vi "HAL camera start acquire.vi"(1 "error in":errorcluster) -> (0 "error out":errorcluster)   [LabVIEW 2011]
doc: "Starts an iXon acquisition (if not already running)"
uses:
  Cascade-specific globals.vi
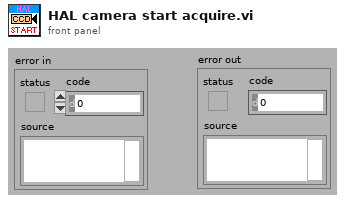
[diagram p1: front panel]
types:
  T1 = cluster{"Camera Handle":u32, "Pulser Handle":u32, "File Handle":u32, "Display Handle":u32, "Image Handle":u32}
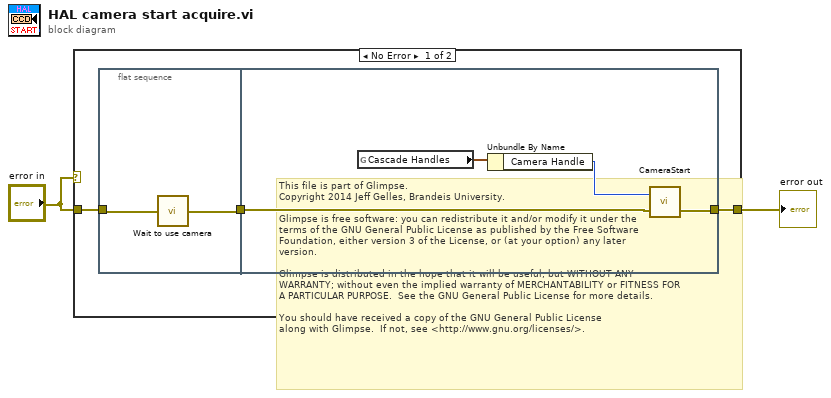
[diagram p0: block diagram]
diagram:
  # "This file is part of Glimpse. \nCopyright 2014 Jeff Gelles, Brandeis University.    \n\nGlimpse is free software: you can redistribute it and/or modify it under the \nterms of the GNU General Public License as published by the Free Software \nFoundation, either version 3 of the License, or (at your option) any later \nversion.\n\nGlimpse is distributed in the hope that it will be useful, but WITHOUT ANY \nWARRANTY; without even the implied warranty of MERCHANTABILITY or FITNESS FOR \nA PARTICULAR PURPOSE.  See the GNU General Public License for more details.\n\nYou should have received a copy of the GNU General Public License\nalong with Glimpse.  If not, see <http://www.gnu.org/licenses/>."
  n1 = case shown="No Error" "error in" {
    tunnel: "error in" -> [w5 w12]
    tunnel: [w4 w12] -> w2
    frame No Error {
      n2 = flat-sequence {
        tunnel: w5 -> [w6]
        tunnel: [w7] -> w3
        tunnel: [w11] -> w4
        tunnel: w3 -> [w8]
        frame #0 {
          n3 = call "Wait to use camera.vi"("error in"=w6) -> ("error out"=w7:errorcluster)
        }
        frame #1 {
          n4 = global read "Cascade-specific globals.vi" "Cascade Handles"() -> (w10:T1)
          n5 = Unbundle By Name(w10) -> ("Camera Handle"=w9:u32)
          n6 = call <userlib>:"CameraStart.vi"("error in"=w8, "Camera Handle"=w9) -> ("error out"=w11:errorcluster)  [unwired: 1 out]
        }
      }
    }
    frame Error {
    }
  }
  "error out" <- w2
